vi "ResetTime.vi"(8 "error in (no error)":errorcluster, 10 "enabled":bool, 11 "SnakeSwitch in":refnum<class "SnakeSwitch.lvclass">) -> (0 "error out":errorcluster, 3 "SnakeSwitch out":refnum<class "SnakeSwitch.lvclass">)   [LabVIEW 2019, in "RT_Game.lvlib" / "SnakeSwitch.lvclass"]
uses:
  SnakeSwitch.lvclass
  SnakeSwitch.lvclass/SnakeSwitch.ctl
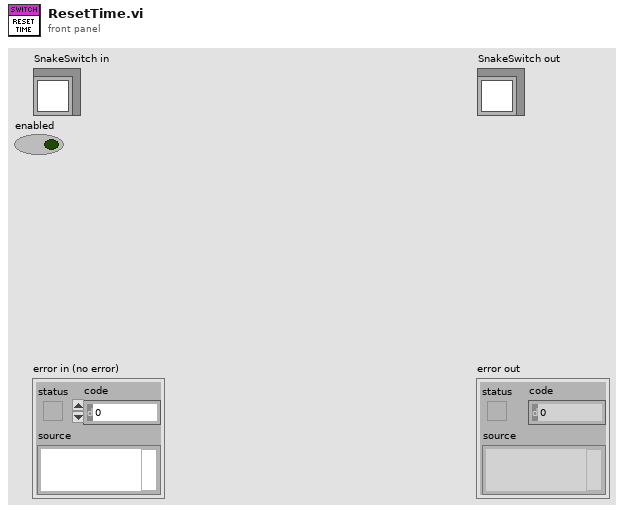
[diagram p1: front panel]
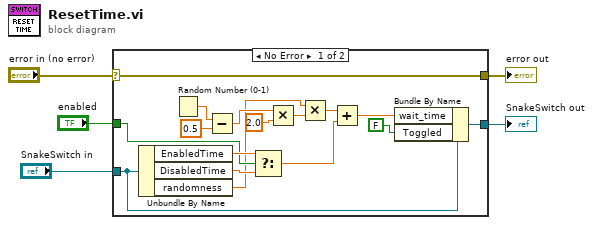
[diagram p0: block diagram]
diagram:
  n1 = case shown="No Error" "error in (no error)" {
    selector: "error in (no error)" -> [w21 w23]
    tunnel: [w21 w23] -> w4
    tunnel: [w16 w22] -> w2
    tunnel: "SnakeSwitch in" -> [w20 w22]
    tunnel: "enabled" -> [w17 _]
    frame No Error {
      n2 = Unbundle By Name(w20) -> ("EnabledTime"=w19:dbl, "DisabledTime"=w18:dbl, "randomness"=w8:dbl)
      n3 = Random Number (0-1)() -> (number: 0 to 1=w13:dbl)
      n4 = Subtract(x=w13, y=0.5) -> (x-y=w11:dbl)
      n5 = Select(t=w19, s=w17, f=w18) -> (s? t:f=w15:dbl)
      n6 = Multiply(x=w11, y=2.0) -> (x*y=w9:dbl)
      n7 = Multiply(x=w8, y=w9) -> (x*y=w7:dbl)
      n8 = Add(x=w7, y=w15) -> (x+y=w14:dbl)
      n9 = Bundle By Name(cluster=w20, "wait_time"=w14, "Toggled"=FALSE) -> (w16:refnum<class "SnakeSwitch.lvclass">)
    }
    frame Error {
    }
  }
  "error out" <- w4
  "SnakeSwitch out" <- w2
